vi "Controller Test Bench (13) - PID.vi"() -> ()   [LabVIEW 2022 SP3]
uses:
  WhiteNoise.ctl
  <vilib>/sound2/lvsound2.llb/Sound Data Format.ctl
  <vilib>/Utility/error.llb/DialogType.ctl
  <vilib>/sound2/lvsound2.llb/Sampling Mode.ctl
  <vilib>/Analysis/4window.llb/windowTd.ctl
  <vilib>/Analysis/3filter.llb/Filter Passband Type.ctl
  <vilib>/DAQmx/read.llb/DAQmx Read (Analog 1D Wfm NChan NSamp).vi
  <vilib>/DAQmx/write.llb/DAQmx Write (Analog Wfm 1Chan NSamp).vi
  <vilib>/addons/control/pid/pid.llb/PID Parameter Manager (DBL Array).vi
  <vilib>/addons/control/pid/pid.llb/PID Derivative Action Buffered (DBL Array).vi
  <vilib>/addons/control/pid/pid.llb/PID Get Advanced Error (DBL Array).vi
  <vilib>/addons/control/pid/pid.llb/PID Integral Action Buffered (DBL Array).vi
  <vilib>/addons/control/pid/pid.llb/PID Resize 1D Array.vi
  <vilib>/addons/control/pid/pid.llb/PID Get Advanced Error (DBL).vi
  <vilib>/sound2/lvsound2.llb/Sound Output Set Volume (Single).vi
  <vilib>/Analysis/3filter.llb/Butterworth Filter (DBL).vi
  <vilib>/sound2/lvsound2.llb/Sound Output Write (DBL Single).vi
  <vilib>/DAQmx/create/channels.llb/DAQmx Create Channel (AI-Acceleration-Accelerometer).vi
  <vilib>/DAQmx/configure/timing.llb/DAQmx Timing (Sample Clock).vi
  <vilib>/DAQmx/configure/task.llb/DAQmx Configure Logging (TDMS).vi
  <vilib>/DAQmx/create/channels.llb/DAQmx Create Channel (AO-Voltage-Basic).vi
  <vilib>/DAQmx/miscellaneous.llb/DAQmx Fill In Error Info.vi
  <vilib>/measure/maspectr.llb/FFT Spectrum (Mag-Phase) for N Chan.vi
  <vilib>/addons/control/pid/pid.llb/PID Advanced (DBL Array).vi
  <vilib>/measure/NI_MAPro.lvlib
  <resource>/objmgr/daqmx.rc
  <vilib>/Analysis/NI_AALPro.lvlib
  <vilib>/measure/NI_MABase.lvlib
  <vilib>/Analysis/NI_AALBase.lvlib
  <vilib>/addons/control/pid/NI_PID_pid.lvlib
panel:
  in  "Sample Rate":dbl=1024.0
  in  "Raw Data":bool
  in  "Active Control":bool
  in  "Folder to save file to":path=path "C:/Users/LAV-UFSC-2023/Documents/LAV-TCC/Dados-Experimentos/Dados-Bancada-LABVIEW"
  in  "Time Out (s)":dbl=60.0
  out "Elapsed Time":i32 caption="Elapsed Time (s)" format="%.2f"
  in  "Tab Control 2":enum32{"Accel0-Only", "Both Accels"}(tab)
  out "Accel0 and Out":waveform(dbl)[](graph)
  out "Accel0, 1 and Out":waveform(dbl)[](graph)
  out "Waveform Graph":waveform(dbl)(graph)
  in  "Output Noise":bool=TRUE
  in  "?":enum32{"White Noise", "Harmonic"}(tab)=enum."Harmonic"
  in  "Cluster":T2={"Seed"=0.0, "Standard Deviation"=1.0, "Reset"=TRUE, "Iterator"=1.0, "Lower Cut-Off 2"=5.0, "Upper Cut-Off 2"=350.0} {"Upper Cut-Off 2" min=5.0 max=350.0 step=10.0; "Lower Cut-Off 2" min=5.0 max=350.0 step=10.0; "Standard Deviation" min=0.001 max=3.5 step=0.05 format="%0.2p"}
  in  "Cluster 2":T3={"Waveform Type"=0, "Frequency"=10.0, "Amplitude"=0.25} {"Frequency" min=5.0 max=350.0 step=10.0 format="%0.2p"; "Waveform Type" items=["Sine Wave", "Triangle Wave", "Square Wave", "Sawtooth Wave"]; "Amplitude" min=0.001 max=0.3 step=0.05 format="%0.2p"}
  in  "Fs":dbl=16384.0
  in  "#s":dbl=360.0
  in  "HW Output Rate":dbl=1000.0 format="%0.2f"
  in  "Tab Control":T4(tab)
  in  "setpoint":dbl[](array[numeric])=[0.0] format="%.2f"
  in  "PID gains":T5(array[cluster])=[{"proportional gain (Kc)"=1.0, "integral time (Ti, min)"=0.01, "derivative time (Td, min)"=0.0}] {"derivative time (Td, min)" format="%.3f"; "integral time (Ti, min)" format="%.3f"; "proportional gain (Kc)" step=0.01 format="%.3f"}
  in  "output range":cluster{"output high":dbl, "output low":dbl}[](array[cluster])=[{"output high"=100.0, "output low"=-100.0}] {"output low" format="%.2f"; "output high" format="%.2f"}
  in  "manual control":dbl[](array[numeric])=[0.0] format="%.2f"
  in  "setpoint range":T6(array[cluster])=[{"setpoint high"=100.0, "setpoint low"=0.0}] {"setpoint high" format="%.2f"; "setpoint low" format="%.2f"}
  in  "Setpoint":dbl
  in  "Gain":dbl min=0.0 step=0.01
  in  "Upper Cut-Off":dbl=400.0
  in  "Lower Cut-Off":dbl=100.0
  out "Phase 2":cluster{"f0":dbl, "df":dbl, "phase":dbl[]}[](graph)
  out "Mag 2":cluster{"f0":dbl, "df":dbl, "magnitude":dbl[]}[](graph)
  in  "FFT":bool=TRUE
  in  "FFT":bool
  in  "Raw Data":bool=TRUE
  # "Data Acquisition"
  # "Log"
  # "Read"
  # "Output"
  # "Filter"
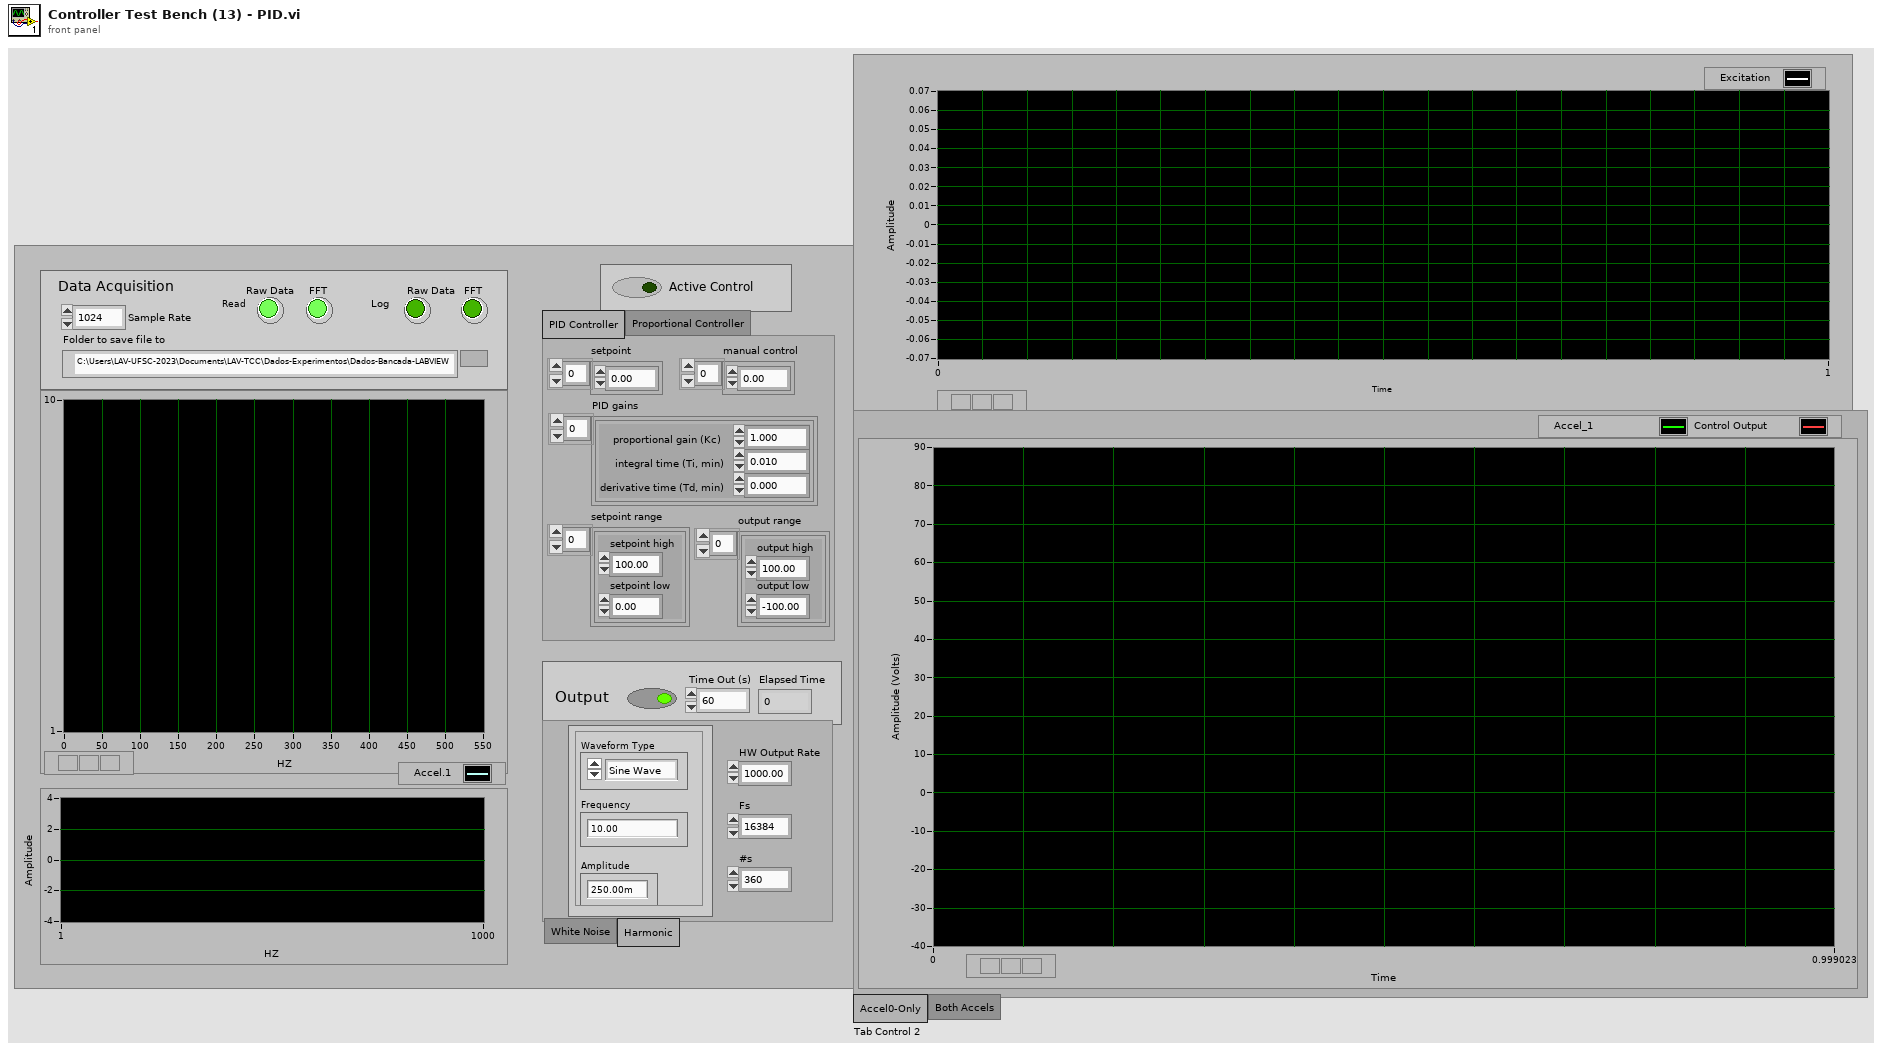
[diagram p1: front panel]
types:
  T1 = typedef "WhiteNoise.ctl" = dbl
  T2 = cluster{"Seed":T1, "Standard Deviation":dbl, "Reset":bool, "Iterator":dbl, "Lower Cut-Off 2":dbl, "Upper Cut-Off 2":dbl}
  T3 = cluster{"Waveform Type":u16, "Frequency":dbl, "Amplitude":dbl}
  T4 = enum32{"PID Controller", "Proportional Controller"}
  T5 = cluster{"proportional gain (Kc)":dbl, "integral time (Ti, min)":dbl, "derivative time (Td, min)":dbl}[]
  T6 = cluster{"setpoint high":dbl, "setpoint low":dbl}[]
  T7 = typedef "Sampling Mode.ctl" = i32
  T8 = typedef "DialogType.ctl" = u16
  T9 = typedef "Sound Data Format.ctl" = cluster{"sample rate (S/s)":dbl, "number of channels":i32, "bits per sample":i32}
  T10 = cluster{"dB On (F)":bool, "unwrap phase (F)":bool, "convert to degree (F)":bool}
  T11 = cluster{"averaging mode":enum16{"No averaging", "Vector averaging", "RMS averaging", "Peak hold"}, "weighting mode":enum16{"Linear", "Exponential"}, "number of averages":u32}
  T12 = typedef "NI_AALPro.lvlib/windowTd.ctl" = u32
  T13 = typedef "Sound Output Task ID.ctl" = u32
  T14 = typedef "NI_AALBase.lvlib/Filter Passband Type.ctl" = enum32{"Lowpass", "Highpass", "Bandpass", "Bandstop"}
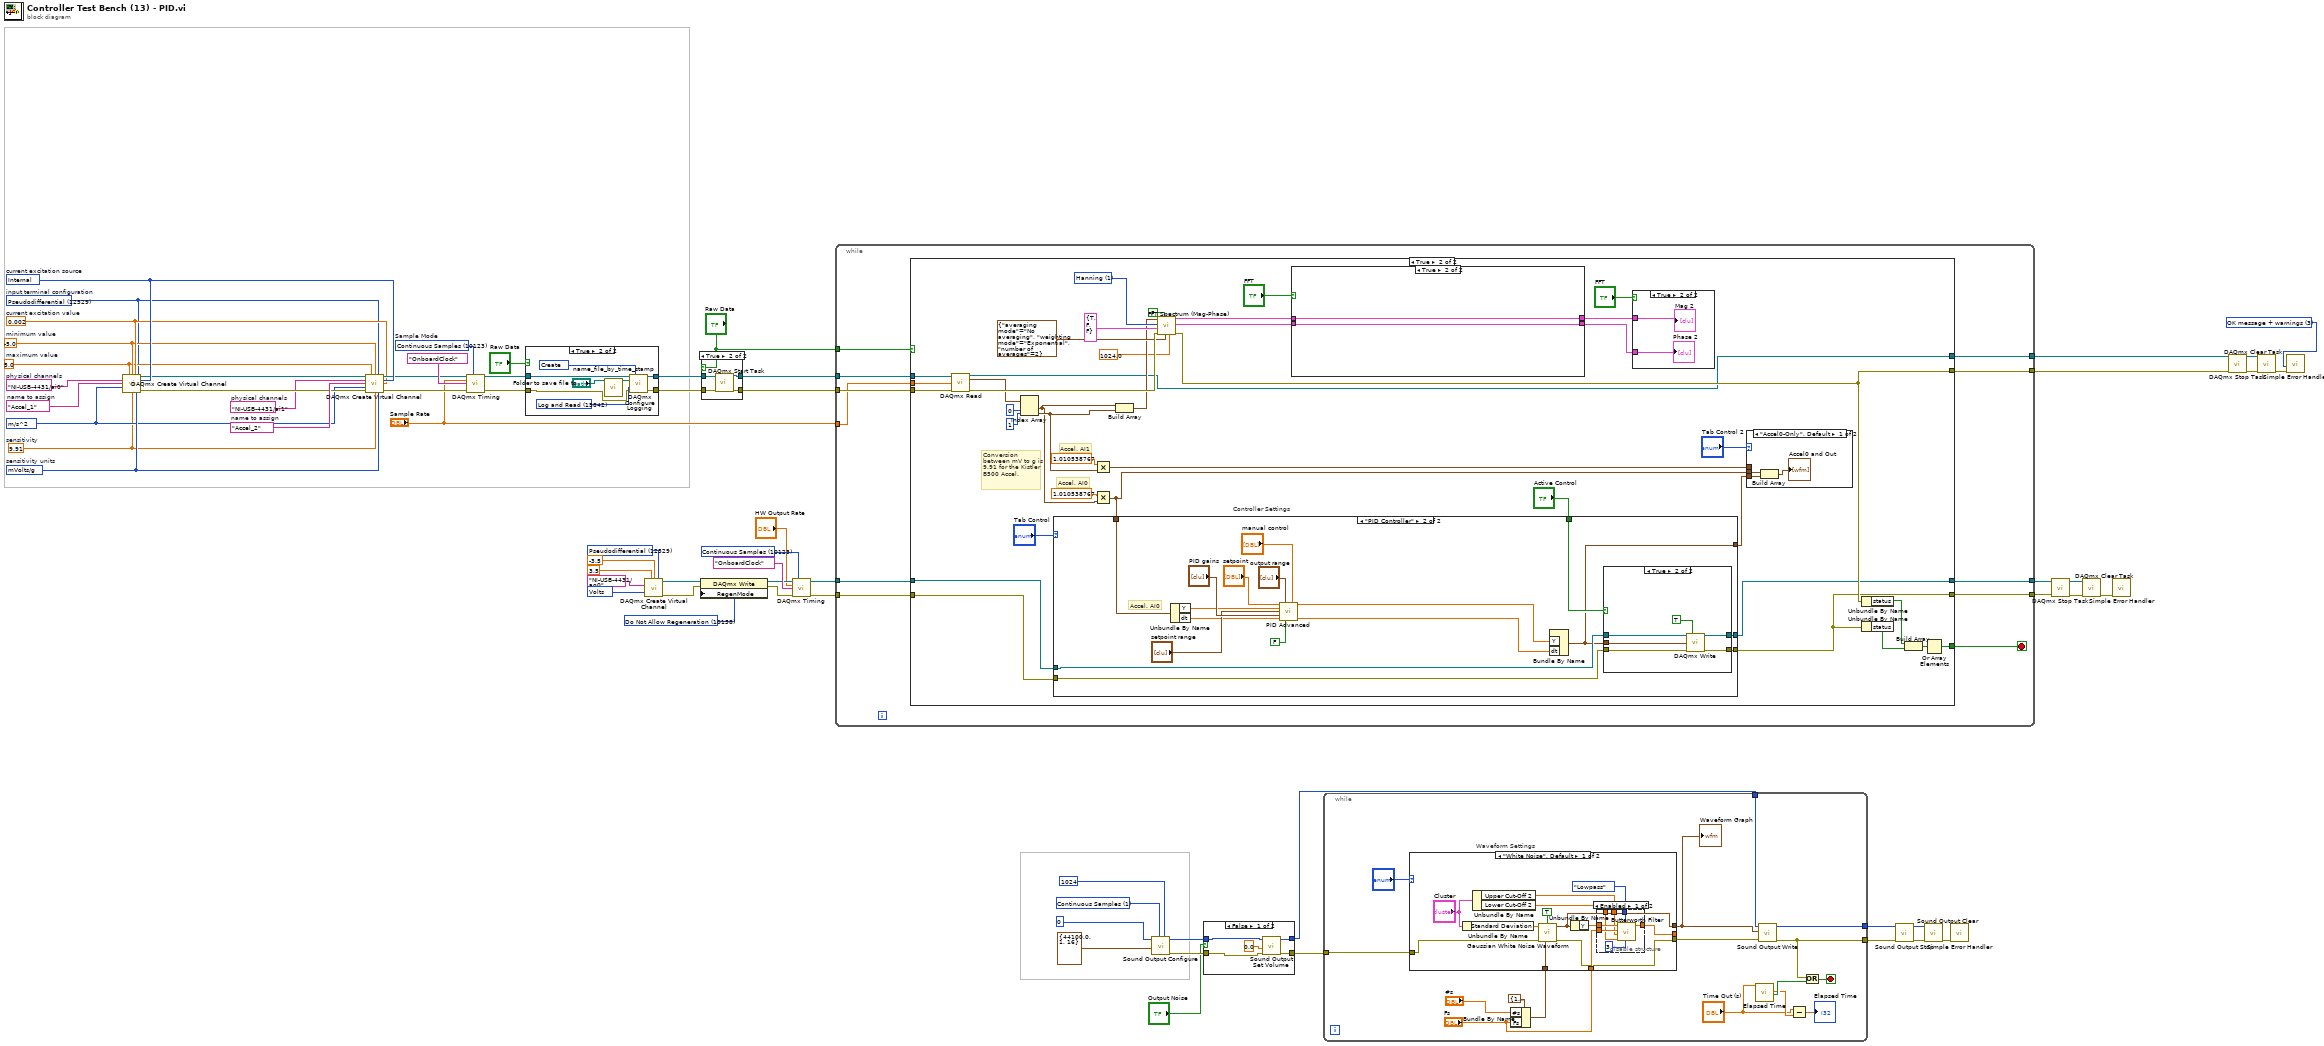
[diagram p0: block diagram]
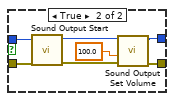
[diagram p2: hidden frame]
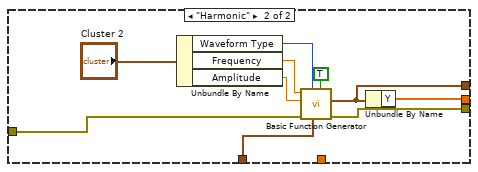
[diagram p4: hidden frame]
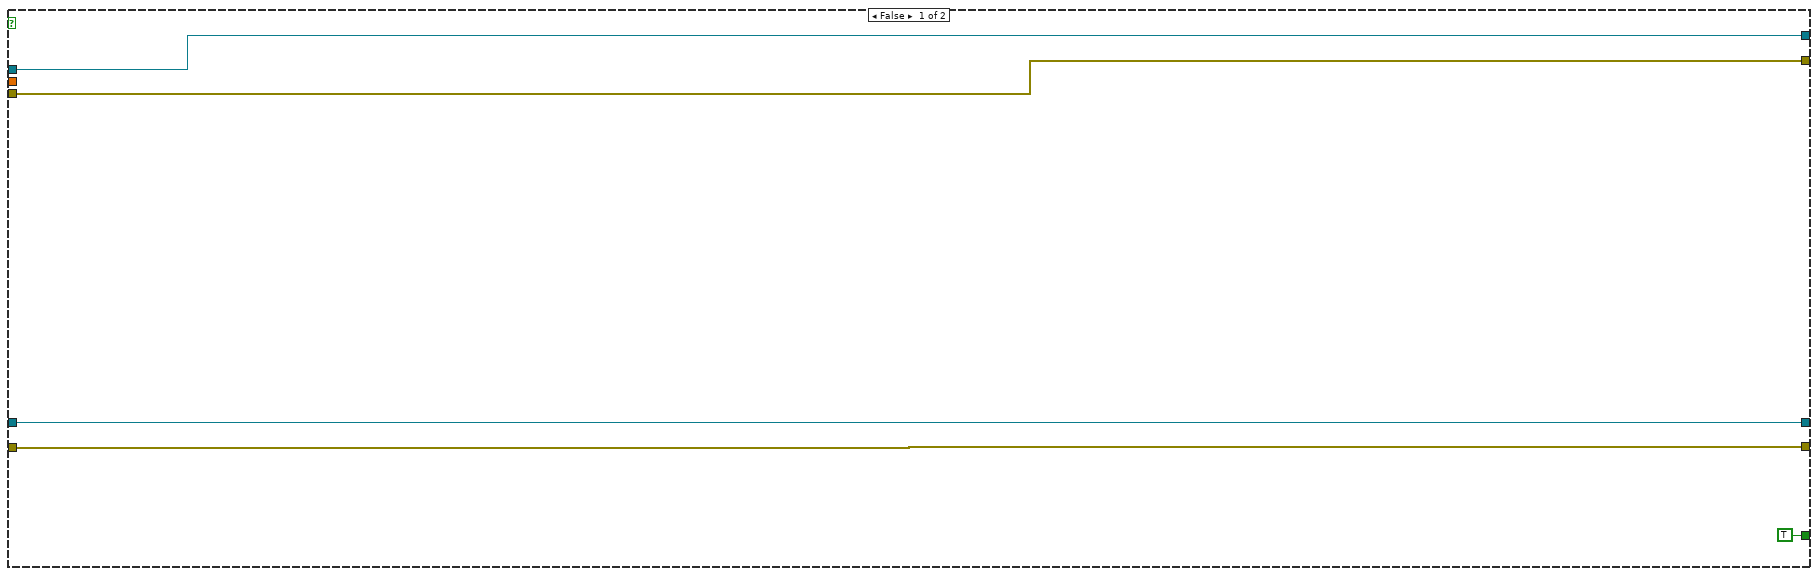
[diagram p5: hidden frame]
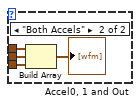
[diagram p6: hidden frame]
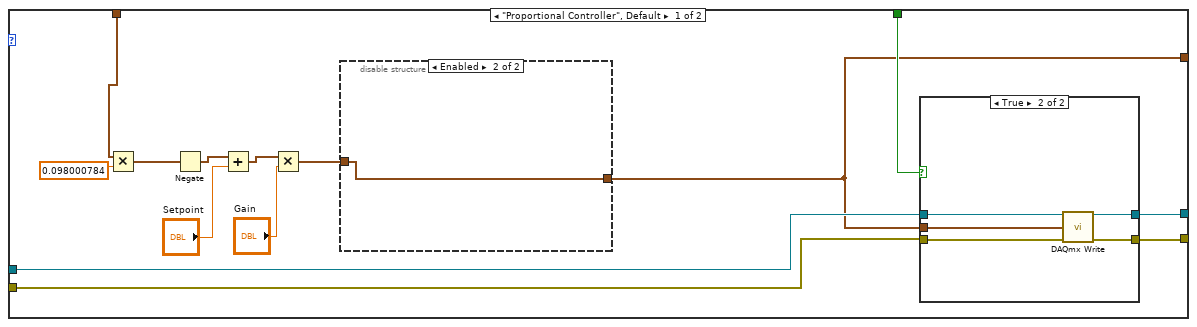
[diagram p7: hidden frame]
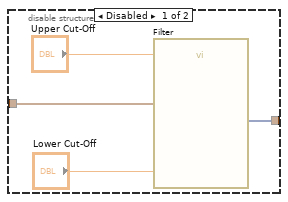
[diagram p8: hidden frame]
diagram:
  w15 = 10123 items=["Finite Samples"=10178, "Continuous Samples"=10123, "Hardware Timed Single Point"=12522] ("sample mode")
  w19 = 10158 items=["Allow Regeneration"=10097, "Do Not Allow Regeneration"=10158] ("RegenMode")
  w24 = 12529 items=["Default"=-1, "RSE"=10083, "Differential"=10106, "Pseudodifferential"=12529] ("output terminal configuration")
  w22 = 10348 items=["Volts"=10348, "From Custom Scale"=10065] ("units")
  w33 = 12470 items=["g"=10186, "m/s^2"=12470, "in/s^2"=12471, "From Custom Scale"=10065] ("units")
  w34 = 12509 items=["mVolts/g"=12509, "Volts/g"=12510]  # sensitivity units
  w32 = 9.91  # sensitivity
  w50 = 0.002  # current excitation value
  w53 = 10200 items=["Internal"=10200, "External"=10167, "None"=10230]  # current excitation source
  w45 = tag "NI-USB-4431/ai0"  # physical channels
  w57 = 10123 items=["Finite Samples"=10178, "Continuous Samples"=10123, "Hardware Timed Single Point"=12522]  # Sample Mode
  w47 = 12529 items=["default"=-1, "RSE"=10083, "NRSE"=10078, "Differential"=10106, "Pseudodifferential"=12529]  # input terminal configuration
  w49 = -5.0  # minimum value
  w48 = 5.0  # maximum value
  w58 = "Accel_1"  # name to assign
  w46 = tag "NI-USB-4431/ai1"  # physical channels
  w55 = "Accel_2"  # name to assign
  w59 = T7 1 items=["Finite Samples", "Continuous Samples"] ("sample mode")
  w60 = T8 3 items=["no dialog", "OK message", "continue or stop message", "OK message + warnings", "continue/stop + warnings"] ("type of dialog (OK msg:1)")
  n1 = call-poly <vilib>:"DAQmx Create Virtual Channel.vi"("maximum value"=w48, "minimum value"=w49, "input terminal configuration"=w47, "physical channels"=w45, "current excitation source"=w53, "name to assign"=w58, "current excitation value"=w50, "units"=w33, "sensitivity"=w32, "sensitivity units"=w34) -> ("task out"=w35:refnum<k21>, "error out"=w54:errorcluster)  [unwired: 4 in]
  n2 = call-poly <vilib>:"DAQmx Create Virtual Channel.vi"("task in"=w35, "maximum value"=w48, "minimum value"=w49, "input terminal configuration"=w47, "physical channels"=w46, "current excitation source"=w53, "name to assign"=w55, "current excitation value"=w50, "units"=w33, "error in"=w54, "sensitivity"=w32, "sensitivity units"=w34) -> ("task out"=w52:refnum<k21>, "error out"=w51:errorcluster)  [unwired: 2 in]
  n3 = call-poly <vilib>:"DAQmx Timing.vi"("task/channels in"=w52, "sample mode"=w57, "rate"="Sample Rate", "source"=tag "OnboardClock" ("Sample Clock Source"), "error in"=w51) -> ("task out"=w31:refnum<k21>, "error out"=w28:errorcluster)  [unwired: 9 in]
  n4 = case shown="True" "Raw Data" {
    tunnel: w31 -> [w69 w74]
    tunnel: [w69 w75] -> w30
    tunnel: [w68 w71] -> w29
    tunnel: w28 -> [w68 w70]
    frame False {
    }
    frame True {
      w76 = 15848 items=["Open"=10437, "Open or Create"=15846, "Create or Replace"=15847, "Create"=15848] ("operation")
      w77 = 15842 items=["Off"=10231, "Log"=15844, "Log and Read"=15842] ("logging mode")
      n5 = call "name_file_by_time_stamp.vi"("Folder to save file to"="Folder to save file to") -> ("New file path"=w73:path)  [unwired: 10 in]
      n6 = call-poly <vilib>:"DAQmx Configure Logging.vi"("task/channels in"=w74, "operation"=w76, "file path"=w73, "logging mode"=w77, "error in"=w70) -> ("task out"=w75:refnum<k21>, "error out"=w71:errorcluster)  [unwired: 9 in]
    }
  }
  n7 = call-poly <vilib>:"DAQmx Create Virtual Channel.vi"("maximum value"=3.5, "minimum value"=-3.5, "output terminal configuration"=w24, "physical channels"=tag "NI-USB-4431/ao0", "units"=w22) -> ("task out"=w18:refnum<k21>, "error out"=w20:errorcluster)  [unwired: 9 in]
  n8 = property class="DAQmx Write"(reference=w18, error in=w20, "RegenMode"=w19) -> (reference out=w16:refnum<k21>, error out=w17:errorcluster)
  n9 = case shown="True" "Raw Data" {
    tunnel: w29 -> [w78 w83]
    tunnel: w30 -> [w79 w82]
    tunnel: [w79 w81] -> w38
    tunnel: [w78 w80] -> w39
    frame False {
    }
    frame True {
      n10 = call <vilib>:"DAQmx Start Task.vi"("task/channels in"=w82, "error in"=w83) -> ("task out"=w81:refnum<k21>, "error out"=w80:errorcluster)  [unwired: 12 in]
    }
  }
  n11 = call-poly <vilib>:"DAQmx Timing.vi"("task/channels in"=w16, "sample mode"=w15, "rate"="HW Output Rate", "source"=tag "OnboardClock" ("Sample Clock Source"), "error in"=w17) -> ("task out"=w6:refnum<k21>, "error out"=w7:errorcluster)  [unwired: 9 in]
  n12 = while {
    tunnel: "Raw Data" -> [w94]
    tunnel: w7 -> [w93]
    tunnel: w39 -> [w92]
    tunnel: w38 -> [w91]
    tunnel: [w90] -> w37
    tunnel: [w89] -> w36
    tunnel: [w88] -> w8
    tunnel: "Sample Rate" -> [w86]
    tunnel: w6 -> [w85]
    tunnel: [w84] -> w5
    stop <- w87 stop-if-true
    n13 = case shown="True" w94 {
      tunnel: w91 -> [w99 w138]
      tunnel: w92 -> [w98 w137]
      tunnel: [w99 w113] -> w89
      tunnel: [w98 w126] -> w90
      tunnel: w93 -> [w97 w122]
      tunnel: [w97 w121] -> w88
      tunnel: [TRUE w120] -> w87
      tunnel: w86 -> [_ w106]
      tunnel: w85 -> [w95 w104]
      tunnel: [w95 w103] -> w84
      frame False {
      }
      frame True {
        w125 = T12 1 items=["Rectangle"=0, "Hanning"=1, "Hamming"=2, "Blackman-Harris"=3, "Exact Blackman"=4, "Blackman"=5, "Flat Top"=6, "4 Term B-Harris "=7, "7 Term B-Harris"=8, "Low Sidelobe"=9, "Blackman Nuttall"=11, "Triangle"=30, "Bartlett-Hanning"=31, "Bohman"=32, "Parzen"=33, "Welch"=34, "Kaiser"=60, "Dolph-Chebyshev"=61, "Gaussian"=62] ("window")
        # "Accel. AI1"
        # "Accel. AI0"
        # "Conversion between mV to g is 9.91 for the Kistler B500 Accel."
        # "Controller Settings"
        n14 = call-poly <vilib>:"DAQmx Read.vi"("task/channels in"=w138, "number of samples per channel"=w106, "error in"=w137) -> ("task out"=w113:refnum<k21>, "data"=w115:waveform(dbl)[], "error out"=w127:errorcluster)  [unwired: 10 in]
        n15 = Index Array(array=w115, index #1=0 ("index"), index #2=1 ("index")) -> (element #1=w109:waveform(dbl), element #2=w110:waveform(dbl))
        n16 = Multiply(x=1.010538767, y=w110) -> (x*y=w108:waveform(dbl))
        n17 = Multiply(x=1.010538767, y=w109) -> (x*y=w101:waveform(dbl))
        n18 = case shown="\"PID Controller\"" "Tab Control" {
          tunnel: w122 -> [w151 w186]
          tunnel: "Active Control" -> [w147 w185]
          tunnel: [w148 w184] -> w121
          tunnel: w101 -> [w152 w180]
          tunnel: w104 -> [w150 w175]
          tunnel: [w149 w174] -> w103
          tunnel: [w146 w172] -> w102
          frame "Proportional Controller", Default {
            n19 = Multiply(x=w152, y=0.098000784) -> (x*y=w154:waveform(dbl))
            n20 = Negate(x=w154) -> (-x=w158:waveform(dbl))
            n21 = Add(x=w158, y="Setpoint") -> (x+y=w157:waveform(dbl))
            n22 = Multiply(x=w157, y="Gain") -> (x*y=w155:waveform(dbl))
            n23 = disable-structure shown="Enabled" {
              disable-tunnel: w155 -> [w163 w164]
              disable-tunnel: [w160 w164] -> w146
              frame Disabled {
                n24 = call "Filter"("Lower Cut-Off"="Lower Cut-Off", "Upper Cut-Off"="Upper Cut-Off", "Signal"=w163) -> ("Filtered Signal"=w160:dynamicdata)  [unwired: 7 in, 1 out]
              }
              frame Enabled {
              }
            }
            n25 = case shown="True" w147 {
              tunnel: w151 -> [w166 w171]
              tunnel: [w166 w170] -> w148
              tunnel: w146 -> [_ w167]
              tunnel: w150 -> [w165 w169]
              tunnel: [w165 w168] -> w149
              frame False {
              }
              frame True {
                n26 = call-poly <vilib>:"DAQmx Write.vi"("task/channels in"=w169, "data"=w167, "error in"=w171) -> ("task out"=w168:refnum<k21>, "error out"=w170:errorcluster)  [unwired: 10 in, 1 out]
              }
            }
          }
          frame "PID Controller" {
            # "Accel. AI0"
            n27 = Unbundle By Name(w180) -> ("Y"=w181:dbl[], "dt"=w177:dbl)
            n28 = call-poly <vilib>:"PID Advanced.vi"("setpoint"="setpoint", "output range"="output range", "manual control"="manual control", "process variable"=w181, "setpoint range"="setpoint range", "PID gains"="PID gains", "dt (s)"=w177, "reinitialize? (F)"=FALSE) -> ("output"=w173:dbl[], "dt out (s)"=w176:dbl)  [unwired: 6 in]
            n29 = Bundle By Name("Y"=w173, "dt"=w176) -> (w172:waveform(dbl))  [unwired: 1 in]
            n30 = case shown="True" w185 {
              tunnel: w186 -> [w190 w196]
              tunnel: [w190 w195] -> w184
              tunnel: w172 -> [_ w194]
              tunnel: w175 -> [w189 w193]
              tunnel: [w189 w192] -> w174
              frame False {
              }
              frame True {
                n31 = call-poly <vilib>:"DAQmx Write.vi"("task/channels in"=w193, "auto start"=TRUE, "data"=w194, "error in"=w196) -> ("task out"=w192:refnum<k21>, "error out"=w195:errorcluster)  [unwired: 9 in, 1 out]
              }
            }
          }
        }
        n32 = Build Array(w109, w110) -> (w114:waveform(dbl)[])
        n33 = call-poly <vilib>:"FFT Spectrum (Mag-Phase).vi"("window parameter"=1024.0, "averaging parameters"=T11 {"averaging mode"=enum."No averaging", "weighting mode"=enum."Exponential", "number of averages"=2}, "restart averaging (F)"=FALSE, "error in (no error)"=w127, "view"=T10 {"dB On (F)"=TRUE, "unwrap phase (F)"=FALSE, "convert to degree (F)"=FALSE}, "window"=w125, "time signals"=w114) -> ("error out"=w126:errorcluster, "phases"=w132:cluster{"f0":dbl, "df":dbl, "phase":dbl[]}[], "magnitudes"=w133:cluster{"f0":dbl, "df":dbl, "magnitude":dbl[]}[])  [unwired: 2 out]
        n34 = case shown="True" "FFT" {
          tunnel: w133 -> [w197 w200]
          tunnel: w132 -> [w198 w199]
          tunnel: [w198 w199] -> w131
          tunnel: [w197 w200] -> w130
          frame False {
          }
          frame True {
          }
        }
        n35 = case shown="True" "FFT" {
          tunnel: w130 -> [_ w202]
          tunnel: w131 -> [_ w201]
          frame False {
          }
          frame True {
            "Mag 2" <- w202
            "Phase 2" <- w201
          }
        }
        n36 = case shown="\"Accel0-Only\", Default" "Tab Control 2" {
          tunnel: w108 -> [_ w145]
          tunnel: w102 -> [w141 w144]
          tunnel: w101 -> [w140 w143]
          frame "Accel0-Only", Default {
            n37 = Build Array(w140, w141) -> (→"Accel0 and Out":waveform(dbl)[])
          }
          frame "Both Accels" {
            n38 = Build Array(w145, w143, w144) -> (→"Accel0, 1 and Out":waveform(dbl)[])
          }
        }
        n39 = Unbundle By Name(w126) -> ("status"=w124:bool)
        n40 = Unbundle By Name(w121) -> ("status"=w129:bool)
        n41 = Build Array(w124, w129) -> (w136:bool[])
        n42 = Or Array Elements(Boolean array=w136) -> (logical OR=w120:bool)
      }
    }
  }
  n43 = call <vilib>:"Sound Output Configure.vi"("number of samples/ch"=1024 ("Number of Samples/ch"), "sample mode"=w59, "sound format"=T9 {"sample rate (S/s)"=44100.0, "number of channels"=1, "bits per sample"=16} ("Sound Format"), "device ID"=u32 0 ("Device ID")) -> ("error out"=w41:errorcluster, "task ID"=w40:T13)  [unwired: 6 in]
  n44 = case shown="False" "Output Noise" {
    tunnel: w41 -> [w206 w214]
    tunnel: w40 -> [w204 w213]
    tunnel: [w205 w209] -> w3
    tunnel: [w203 w208] -> w2
    frame False {
      n45 = call-poly <vilib>:"Sound Output Set Volume.vi"("error in (no error)"=w206, "volume"=0.0, "task ID"=w204) -> ("error out"=w205:errorcluster, "task ID out"=w203:T13)  [unwired: 7 in]
    }
    frame True {
      n46 = call <vilib>:"Sound Output Start.vi"("error in (no error)"=w214, "task ID"=w213) -> ("error out"=w212:errorcluster, "task ID out"=w210:T13)  [unwired: 8 in]
      n47 = call-poly <vilib>:"Sound Output Set Volume.vi"("error in (no error)"=w212, "volume"=100.0, "task ID"=w210) -> ("error out"=w209:errorcluster, "task ID out"=w208:T13)  [unwired: 7 in]
    }
  }
  n48 = while {
    tunnel: w3 -> [w223]
    tunnel: [w222] -> w10
    tunnel: w2 -> [w217]
    tunnel: [w215] -> w9
    stop <- w228 stop-if-true
    # "Waveform Settings"
    n49 = Bundle By Name(cluster=cluster{"Fs":dbl, "#s":dbl} {"Fs"=1000.0, "#s"=1000.0} ("sampling info"), "#s"="#s", "Fs"="Fs") -> (w220:cluster{"Fs":dbl, "#s":dbl})
    n50 = case shown="\"White Noise\", Default" "?" {
      tunnel: w220 -> [w243 w260]
      tunnel: w223 -> [w242 w261]
      tunnel: [w232 w259] -> w229
      tunnel: [w233 w253] -> _
      tunnel: "Fs" -> [w236 _]
      tunnel: [w231 w252] -> w216
      frame "White Noise", Default {
        n51 = Unbundle By Name("Cluster") -> ("Standard Deviation"=w239:dbl)
        n52 = Unbundle By Name("Cluster") -> ("Upper Cut-Off 2"=w234:dbl, "Lower Cut-Off 2"=w235:dbl)
        n53 = call <vilib>:"Gaussian White Noise Waveform.vi"("sampling info"=w243, "reset signal"=TRUE, "error in (no error)"=w242, "standard deviation"=w239) -> ("error out"=w232:errorcluster, "signal out"=w231:waveform(dbl))  [unwired: 6 in]
        n54 = Unbundle By Name(w231) -> ("Y"=w237:dbl[])
        n55 = disable-structure shown="Enabled" {
          disable-tunnel: Filter_Passband_Type."Lowpass" ("filter type") -> [w250 _]
          disable-tunnel: w237 -> [w249 w251]
          disable-tunnel: w236 -> [w248 _]
          disable-tunnel: w235 -> [w247 _]
          disable-tunnel: w234 -> [w246 _]
          disable-tunnel: [w244 w251] -> w233
          frame Enabled {
            n56 = call-poly <vilib>:"Butterworth Filter.vi"("order"=3, "filter type"=w250, "low cutoff freq: fl"=w247, "high cutoff freq: fh"=w246, "sampling freq: fs"=w248, "X"=w249) -> ("Filtered X"=w244:dbl[])  [unwired: 2 in, 1 out]
          }
          frame Disabled {
          }
        }
      }
      frame "Harmonic" {
        n57 = Unbundle By Name("Cluster 2") -> ("Waveform Type"=w257:u16, "Frequency"=w256:dbl, "Amplitude"=w255:dbl)
        n58 = call <vilib>:"Basic Function Generator.vi"("reset signal"=TRUE, "sampling info"=w260, "signal type"=w257, "error in (no error)"=w261, "amplitude"=w255, "frequency"=w256) -> ("error out"=w259:errorcluster, "signal out"=w252:waveform(dbl))  [unwired: 3 in, 1 out]
        n59 = Unbundle By Name(w252) -> ("Y"=w253:dbl[])
      }
    }
    "Waveform Graph" <- w216
    n60 = call "Elapsed Time"("Time Target (s)"="Time Out (s)") -> ("Elapsed Time (s)"=w225:dbl, "Time has Elapsed"=w226:bool)  [unwired: 11 in, 6 out]
    n61 = call-poly <vilib>:"Sound Output Write.vi"("error in (no error)"=w229, "data"=w216, "task ID"=w217) -> ("error out"=w222:errorcluster, "task ID out"=w215:T13)  [unwired: 7 in]
    n62 = Subtract(x="Time Out (s)", y=w225) -> (x-y=→"Elapsed Time":dbl)
    n63 = Or(x=w222, y=w226) -> (x .or. y?=w228:bool)
  }
  n64 = call <vilib>:"Sound Output Stop.vi"("error in (no error)"=w10, "task ID"=w9) -> ("error out"=w44:errorcluster, "task ID out"=w43:T13)  [unwired: 8 in]
  n65 = call <vilib>:"Sound Output Clear.vi"("error in (no error)"=w44, "task ID"=w43) -> ("error out"=w42:errorcluster)  [unwired: 9 in]
  n66 = call <vilib>:"Simple Error Handler.vi"("error in (no error)"=w42) -> ()  [unwired: 4 in, 5 out]
  n67 = call <vilib>:"DAQmx Stop Task.vi"("task/channels in"=w5, "error in"=w8) -> ("task out"=w14:refnum<k21>, "error out"=w13:errorcluster)  [unwired: 12 in]
  n68 = call <vilib>:"DAQmx Clear Task.vi"("task in"=w14, "error in"=w13) -> ("error out"=w12:errorcluster)  [unwired: 13 in]
  n69 = call <vilib>:"Simple Error Handler.vi"("error in (no error)"=w12) -> ()  [unwired: 4 in, 5 out]
  n70 = call <vilib>:"DAQmx Stop Task.vi"("task/channels in"=w36, "error in"=w37) -> ("task out"=w63:refnum<k21>, "error out"=w62:errorcluster)  [unwired: 12 in]
  n71 = call <vilib>:"DAQmx Clear Task.vi"("task in"=w63, "error in"=w62) -> ("error out"=w64:errorcluster)  [unwired: 13 in]
  n72 = call <vilib>:"Simple Error Handler.vi"("type of dialog (OK msg:1)"=w60, "error in (no error)"=w64) -> ()  [unwired: 3 in, 5 out]
